vi "语音识别正确跳出信息.vi"() -> (1 "Boolean":bool)   [LabVIEW 2023]
uses:
  <vilib>/Utility/file.llb/Read From Spreadsheet File (string).vi
  global_variable.vi
panel:
  out "出入时间":string
  out "图片显示":picture
  in  "?":bool
  out "录入时间":string
  out "联系电话":string
  out "学院":string
  out "寝室号":string
  out "学号":string
  out "姓名":string
  # "通过门禁检测"
  # "通过门禁检测"
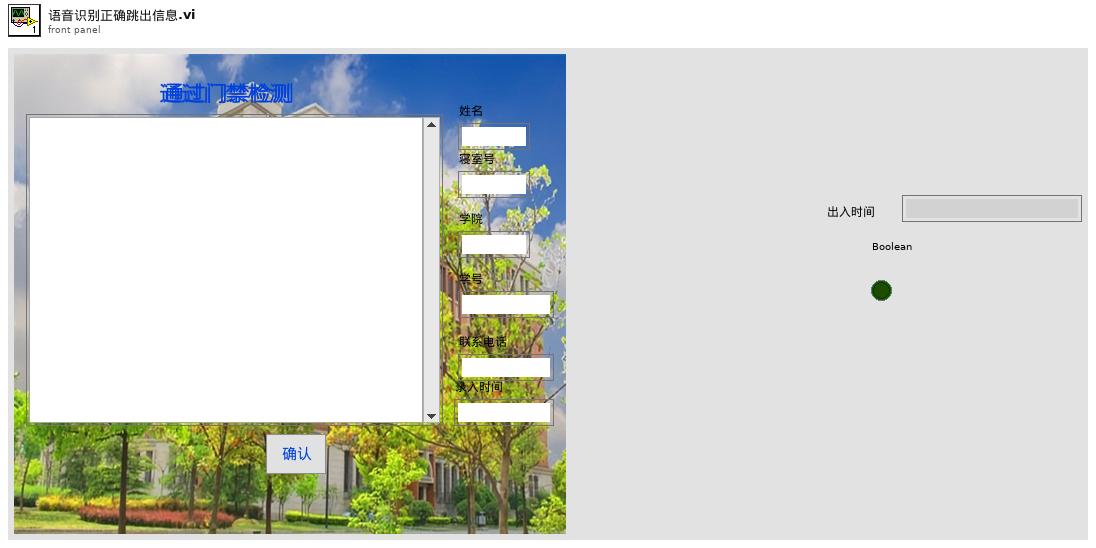
[diagram p1: front panel]
types:
  T1 = enum16{"open", "replace", "create", "open or create", "replace or create", "replace or create with confirmation"}
  T2 = cluster{"all rows[0]":string, "all rows[1]":string, "all rows[2]":string, "all rows[3]":string, "all rows[4]":string, "all rows[5]":string, "all rows[6]":string, "all rows[7]":string, "all rows[8]":string}
  T3 = typedef "imagedata.ctl" = cluster{"image type":i32, "image depth":i32, "image":u8[], "mask":u8[], "colors":u32[], "Rectangle":cluster{"left":i16, "top":i16, "right":i16, "bottom":i16}}
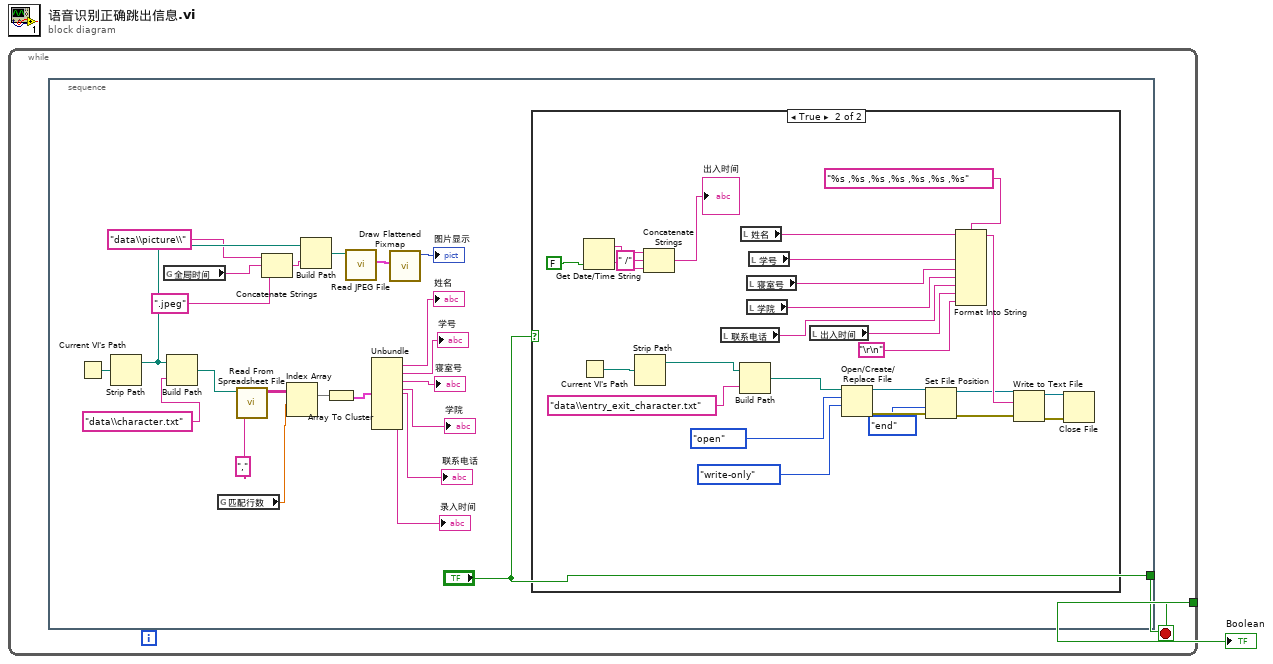
[diagram p0: block diagram]
diagram:
  n1 = while {
    tunnel: [w2] -> w1
    stop <- w2 stop-if-true
    n2 = stacked-sequence {
      tunnel: ["?"] -> w2
      frame #0 {
        n3 = Current VI's Path() -> (path=w25:path)
        n4 = Strip Path(path=w25) -> (stripped path=w11:path)  [unwired: 1 out]
        n5 = global read "global_variable.vi" "全局时间"() -> (w8:string)
        n6 = Build Path(base path=w11, name or relative path="data\\character.txt") -> (appended path=w22:path)
        n7 = global read "global_variable.vi" "匹配行数"() -> (w12:dbl)
        n8 = call-poly <vilib>:"Read From Spreadsheet File.vi"("delimiter (\\t)"=",", "file path (dialog if empty)"=w22) -> ("all rows"=w21:string[][])  [unwired: 5 in, 4 out]
        n9 = Concatenate Strings("data\\picture\\" ("string"), w8, ".jpeg" ("string")) -> (w7:string)
        n10 = Index Array(array=w21, index (row)=w12) -> (element=w20:string[])  [unwired: 1 in]
        n11 = Build Path(base path=w11, name or relative path=w7) -> (appended path=w6:path)
        n12 = Array To Cluster(array=w20) -> (cluster=w19:T2)
        n13 = call <vilib>:"Read JPEG File.vi"("path to JPEG file"=w6) -> ("image data"=w5:T3)  [unwired: 8 in, 2 out]
        n14 = Unbundle(w19) -> ("all rows[0]"=→"姓名":string, "all rows[1]"=→"学号":string, "all rows[2]"=→"寝室号":string, "all rows[3]"=→"学院":string, "all rows[4]"=→"联系电话":string, "all rows[6]"=→"录入时间":string)  [unwired: 3 out]
        n15 = call <vilib>:"Draw Flattened Pixmap.vi"("image data"=w5) -> ("new picture"=→"图片显示":picture)  [unwired: 8 in]
        n16 = case shown="True" "?" {
          frame False {
          }
          frame True {
            n17 = Current VI's Path() -> (path=w52:path)
            n18 = Get Date/Time String(want seconds? (F)=FALSE) -> (date string=w29:string, time string=w27:string)  [unwired: 2 in]
            n19 = Strip Path(path=w52) -> (stripped path=w51:path)  [unwired: 1 out]
            n20 = Concatenate Strings(w29, " /" ("string"), w27) -> (→"出入时间":string)
            n21 = local read "联系电话"() -> (w38:string)
            n22 = Build Path(base path=w51, name or relative path="data\\entry_exit_character.txt") -> (appended path=w50:path)
            n23 = local read "姓名"() -> (w42:string)
            n24 = local read "寝室号"() -> (w40:string)
            n25 = local read "学院"() -> (w39:string)
            n26 = local read "学号"() -> (w41:string)
            n27 = local read "出入时间"() -> (w37:string)
            n28 = Open/Create/Replace File(file path (use dialog)=w50, operation (0:open)=T1."open", access (0:read/write)=enum16{"read/write", "read-only", "write-only"}."write-only") -> (refnum out=w46:refnum<file>, error out=w44:errorcluster)  [unwired: 3 in, 1 out]
            n29 = Set File Position(refnum=w46, from (0:start)=enum16{"start", "end", "current"}."end", error in=w44) -> (refnum out=w45:refnum<file>, error out=w43:errorcluster)  [unwired: 1 in]
            n30 = Format Into String(format string="%s ,%s ,%s ,%s ,%s ,%s ,%s", w42, w41, w40, w39, w38, w37, "\r\n") -> (resulting string=w49:string)  [unwired: 2 in, 1 out]
            n31 = Write to Text File(file (use dialog)=w45, text=w49, error in=w43) -> (refnum out=w47:refnum<file>, error out=w48:errorcluster)  [unwired: 1 in, 1 out]
            n32 = Close File(refnum=w47, error in=w48) -> ()  [unwired: 2 out]
          }
        }
      }
    }
  }
  "Boolean" <- w1
